vi "Make Default Model.vi"(8 "error in (no error)":errorcluster) -> (0 "error out":errorcluster, 3 "Result Model out":refnum<class "Result Model.lvclass">)   [LabVIEW 2020, in "Result Model Result Recording Test.lvclass"]
uses:
  Result Model Result Recording Test.lvclass
  source/User Interface/Result Model/Result Model.lvclass
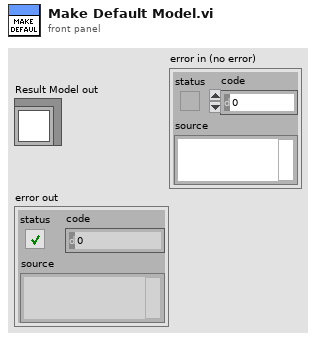
[diagram p1: front panel]
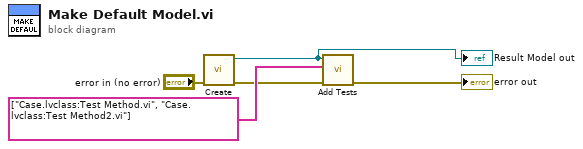
[diagram p0: block diagram]
diagram:
  n1 = call "Create.vi"("error in (no error)"="error in (no error)") -> ("error out"=w2:errorcluster, "Result Model out"=w4:refnum<class "Result Model.lvclass">)  [unwired: 9 in]
  "Result Model out" <- w4
  n2 = call "Add Tests.vi"("error in (no error)"=w2, "Tests"=string[] ["Case.lvclass:Test Method.vi", "Case.lvclass:Test Method2.vi"], "Result Model by Reference In"=w4) -> ("error out"=→"error out":errorcluster)  [unwired: 8 in]
